vi "Get Relay Task Name.vi"(8 "error in (no error)":errorcluster, 11 "Config Data":T1={"Diagnostic_Modes"={"Selected_Mode"=""}, "Basic_Health"={"Task_Name"="", "Sample_Rate_Hz"=0.0, "Samples_Per_Channel"=0}, "Complex_Machinery"={"Task_Name"="", "Sample_Rate_Hz"=0.0, "Samples_Per_Channel"=0}, "Multi_Point"={"Task_Name"="", "Sample_Rate_Hz"=0.0, "Samples_Per_Channel"=0}, "System_Settings"={"Simulation_Mode "="", "Options"=enum."Healthy"}, "Relay"={"Task_Name"="Local_Trip_Relay_Task"}}) -> (0 "error out":errorcluster, 3 "Relay Task Name":string)   [LabVIEW 2026, in "Acquisition.lvlib"]
uses:
  Acquisition.lvlib
  Controls/Vibration_Monitor_Config.ctl
  Controls/Vibration_Profile.ctl
  Controls/System_Settings.ctl
  Controls/Options.ctl
  Controls/Relay_Profile.ctl
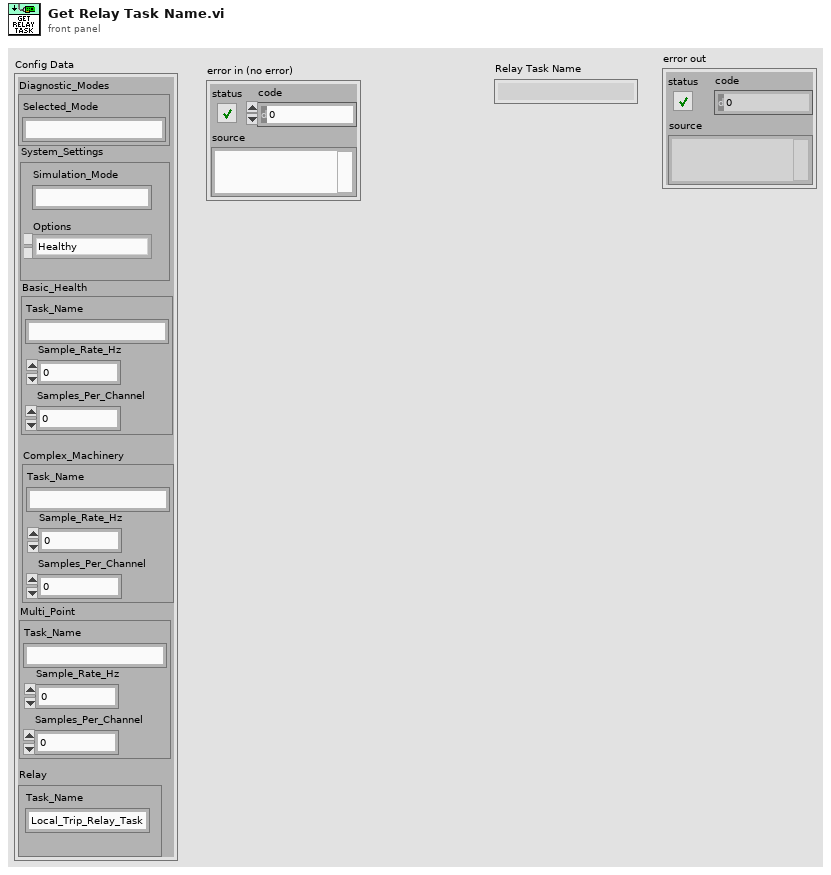
[diagram p1: front panel]
types:
  T1 = typedef "Vibration_Monitor_Config.ctl" = cluster{"Diagnostic_Modes":cluster{"Selected_Mode":string}, "Basic_Health":T2, "Complex_Machinery":T2, "Multi_Point":T2, "System_Settings":T3, "Relay":T5}
  T2 = typedef "Vibration_Profile.ctl" = cluster{"Task_Name":string, "Sample_Rate_Hz":dbl, "Samples_Per_Channel":i32}
  T3 = typedef "System_Settings.ctl" = cluster{"Simulation_Mode ":string, "Options":T4}
  T4 = typedef "Options.ctl" = enum16{"Healthy", "Unbalance_Alert", "Bearing_Fault_Critical", "Sweep_Test"}
  T5 = typedef "Relay_Profile.ctl" = cluster{"Task_Name":string}
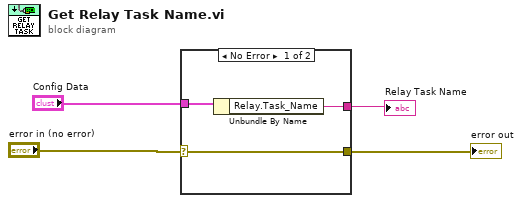
[diagram p0: block diagram]
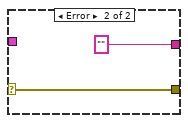
[diagram p2: hidden frame]
diagram:
  n1 = case shown="No Error" "error in (no error)" {
    selector: "error in (no error)" -> [w7 w8]
    tunnel: [w7 w8] -> w3
    tunnel: "Config Data" -> [w6 _]
    tunnel: [w5 "" ("Task_Name")] -> w1
    frame No Error {
      n2 = Unbundle By Name(w6) -> ("Relay.Task_Name"=w5:string)
    }
    frame Error {
    }
  }
  "error out" <- w3
  "Relay Task Name" <- w1
